vi "Expand Special Cluster.vi"(6 "Special Term Indices In":T1={"Action"=-1, "Init"=-1, "Tag"=-1, "State in"=-1, "State out"=-1, "Error"=-1}, 9 "Initial Type Descriptor":T2, 10 "Special Terminal":T6, 11 "Variant":variant) -> (0 "Save Types?":bool, 1 "Contained Types":T2[](array[typedef]), 4 "Special Term Indices":T1)   [LabVIEW 2020, in "FlexBlock.xnode"]
uses:
  FlexBlock.xnode
  FlexBlocks/Special Terminal.ctl
  FlexBlocks/Type Descriptor.ctl
  FlexBlocks/Terminal Direction.ctl
  FlexBlocks/Value Mode.ctl
  FlexBlocks/Terminal State.ctl
  FlexBlocks/Special Terminal Indices.ctl
  <vilib>/addons/analyzer/_analyzerutils.llb/VIAnUtil Check Type If ErrClust.vi
  <vilib>/Utility/Data Type/NI_Data Type.lvlib
  FlexBlocks/FlexBlocks.lvlib
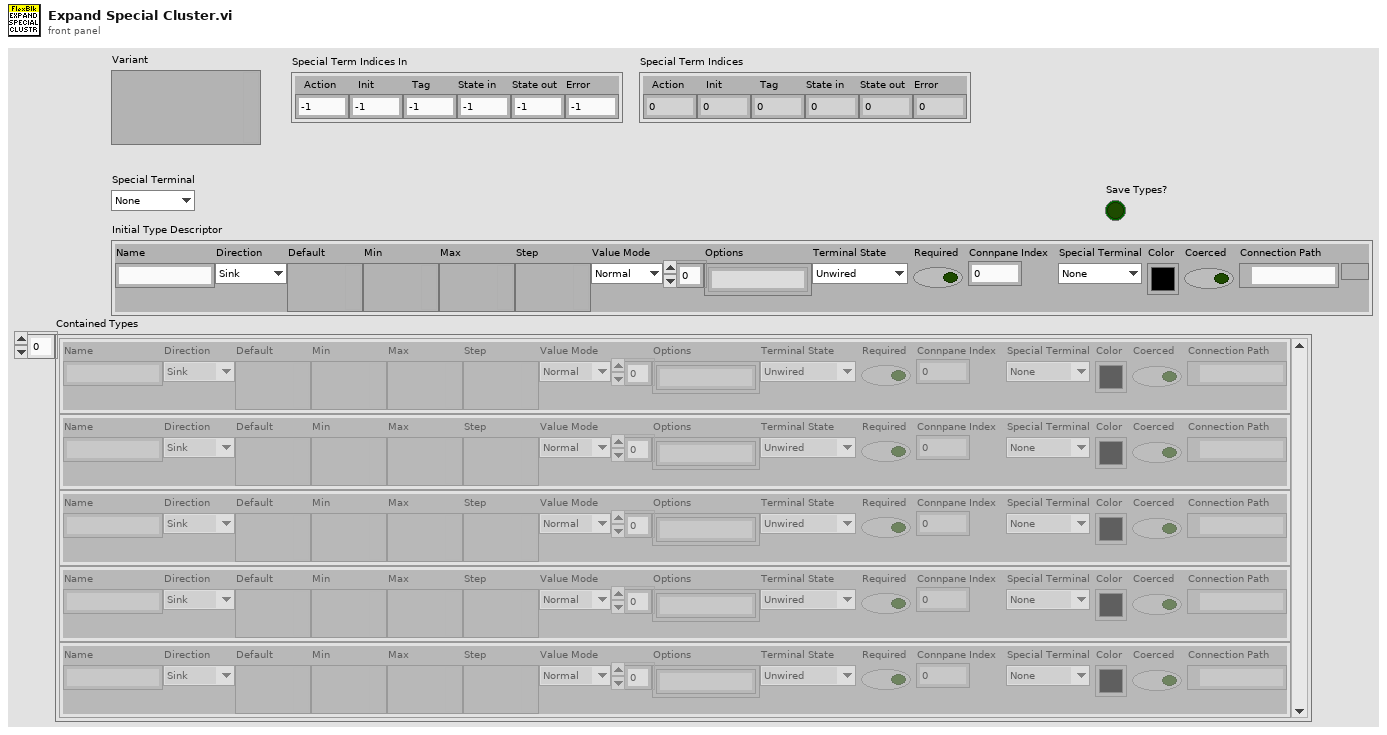
[diagram p1: front panel]
types:
  T1 = typedef "FlexBlocks.lvlib/Special Terminal Indices.ctl" = cluster{"Action":i32, "Init":i32, "Tag":i32, "State in":i32, "State out":i32, "Error":i32}
  T2 = typedef "FlexBlocks.lvlib/Type Descriptor.ctl" = cluster{"Name":string, "Direction":T3, "Default":variant, "Min":variant, "Max":variant, "Step":variant, "Value Mode":T4, "Options":string[], "Terminal State":T5, "Required":bool, "Connpane Index":i32, "Special Terminal":T6, "Color":u32, "Coerced":bool, "Connection Path":path}
  T3 = typedef "FlexBlocks.lvlib/Terminal Direction.ctl" = enum16{"Sink", "Source"}
  T4 = typedef "FlexBlocks.lvlib/Value Mode.ctl" = enum16{"Normal", "Range", "Select"}
  T5 = typedef "FlexBlocks.lvlib/Terminal State.ctl" = enum16{"Unwired", "BadType", "BadRef", "Channel", "Value", "Control Ref"}
  T6 = typedef "FlexBlocks.lvlib/Special Terminal.ctl" = enum16{"None", "Action", "Init", "Tag", "State in", "State out", "Error"}
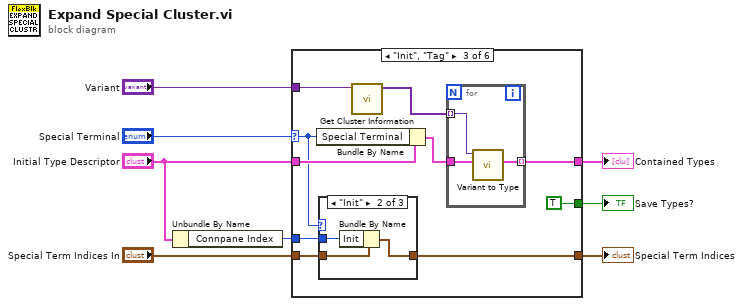
[diagram p0: block diagram]
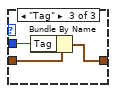
[diagram p5: hidden frame]
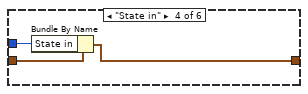
[diagram p6: hidden frame]
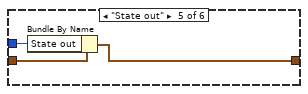
[diagram p7: hidden frame]
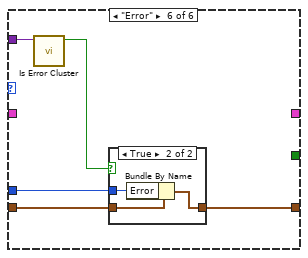
[diagram p8: hidden frame]
diagram:
  n1 = Unbundle By Name("Initial Type Descriptor") -> ("Connpane Index"=w5:i32)
  n2 = case shown="\"Init\", \"Tag\"" "Special Terminal" {
    selector: "Special Terminal" -> [_ _ w17 _ _ _]
    tunnel: "Initial Type Descriptor" -> [_ _ w19 _ _ _]
    tunnel: "Variant" -> [_ _ w18 _ _ w38]
    tunnel: w5 -> [_ _ w14 w32 w35 w40]
    tunnel: "Special Term Indices In" -> [w9 w10 w13 w33 w36 w41]
    tunnel: [_ _ TRUE _ _ _] -> w3
    tunnel: [w9 w10 w12 w31 w34 w39] -> w2
    tunnel: [_ _ w11 _ _ _] -> w1
    frame "None" {
    }
    frame "Action" {
    }
    frame "Init", "Tag" {
      n3 = Bundle By Name(cluster=w19, "Special Terminal"=w17) -> (w16:T2)
      n4 = case shown="\"Init\"" w17 {
        tunnel: w14 -> [_ w26 w29]
        tunnel: w13 -> [w24 w27 w30]
        tunnel: [w24 w25 w28] -> w12
        frame Default {
        }
        frame "Init" {
          n5 = Bundle By Name(cluster=w27, "Init"=w26) -> (w25:T1)
        }
        frame "Tag" {
          n6 = Bundle By Name(cluster=w30, "Tag"=w29) -> (w28:T1)
        }
      }
      n7 = call <vilib>:"Get Cluster Information.vi"("variant"=w18) -> ("cluster elements"=w15:variant[])  [unwired: 9 in, 1 out]
      n8 = for {
        tunnel: w16 -> [w23]
        tunnel: w15 -> [w21] mode=indexing
        tunnel: [w22] -> w11 mode=indexing
        n9 = call "Variant to Type.vi"("Type In"=w23, "Value"=w21) -> ("Type"=w22:T2)  [unwired: 9 in]
      }
    }
    frame "State in" {
      n10 = Bundle By Name(cluster=w33, "State in"=w32) -> (w31:T1)
    }
    frame "State out" {
      n11 = Bundle By Name(cluster=w36, "State out"=w35) -> (w34:T1)
    }
    frame "Error" {
      n12 = call <vilib>:"Is Error Cluster.vi"("variant"=w38) -> ("is error cluster?"=w37:bool)  [unwired: 9 in, 1 out]
      n13 = case shown="True" w37 {
        tunnel: w41 -> [w42 w45]
        tunnel: w40 -> [_ w44]
        tunnel: [w42 w43] -> w39
        frame False {
        }
        frame True {
          n14 = Bundle By Name(cluster=w45, "Error"=w44) -> (w43:T1)
        }
      }
    }
  }
  "Contained Types" <- w1
  "Save Types?" <- w3
  "Special Term Indices" <- w2
